vi "SSP - set cluster element.vi"(8 "error in (no error)":errorcluster, 11 "JSON string":string) -> (0 "error out":errorcluster, 3 "value":string)   [LabVIEW 2020, in "ui-testing.lvlib"]
doc: "copyright: Thomas Zilliox©"
uses:
  ui-testing.lvlib
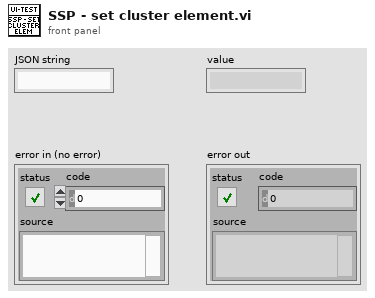
[diagram p1: front panel]
types:
  T1 = cluster{"name":string, "type":string, "value":string, "layers":string[], "subpanel":string, "subsubpanel":string}
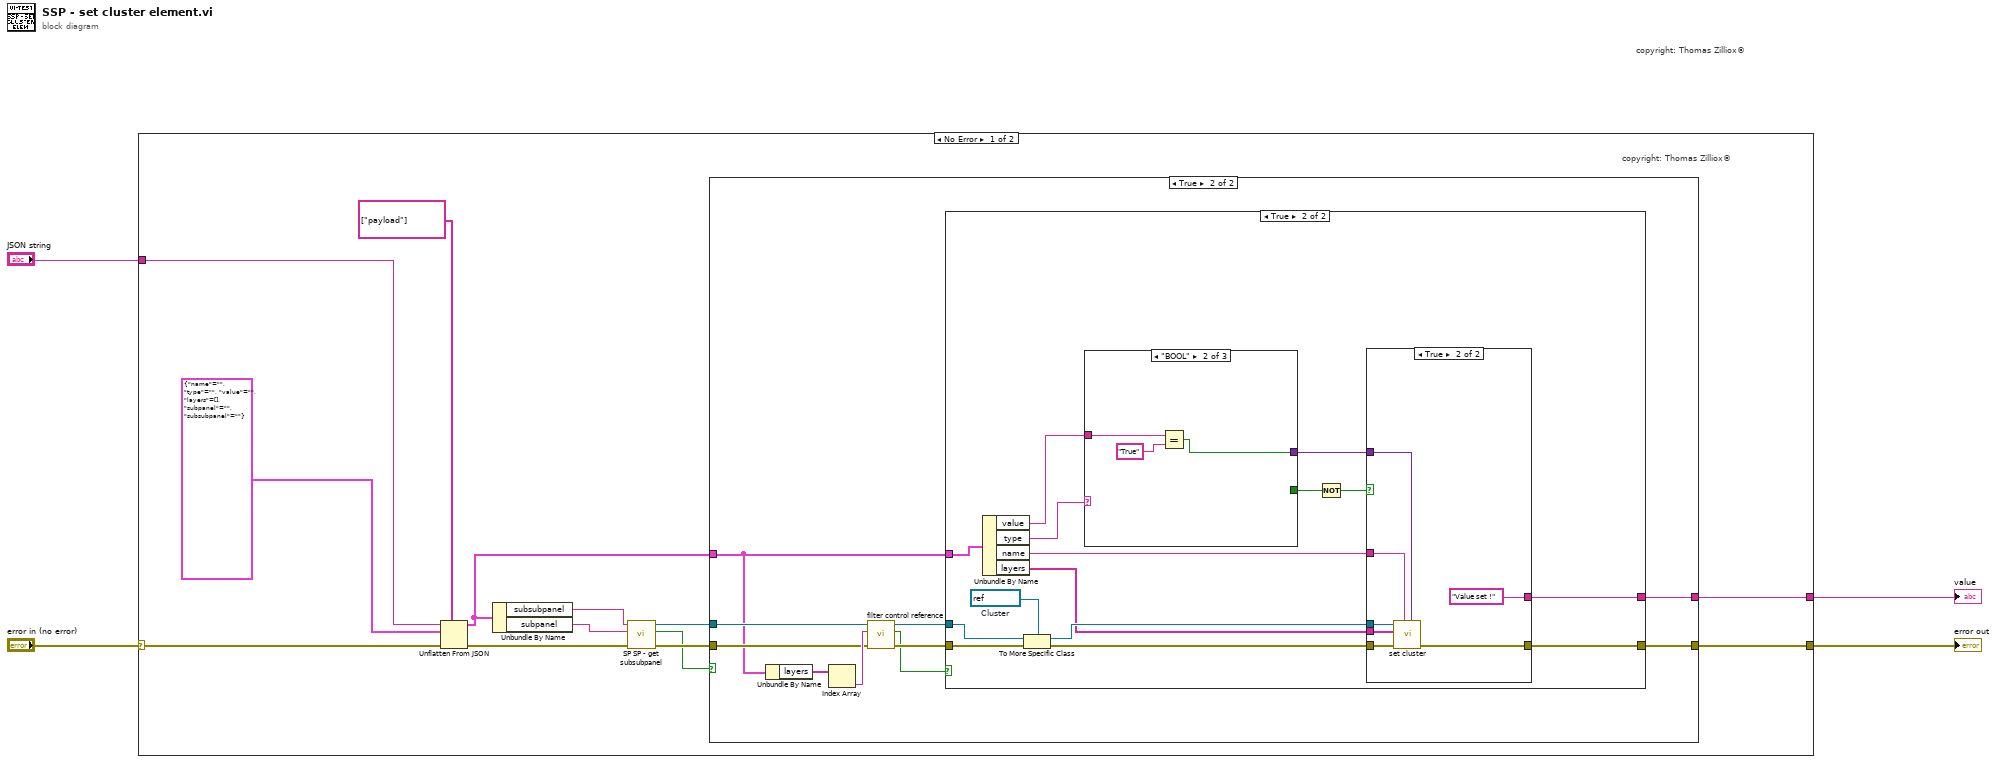
[diagram p0: block diagram]
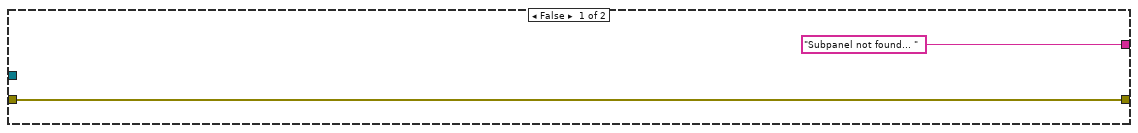
[diagram p2: hidden frame]
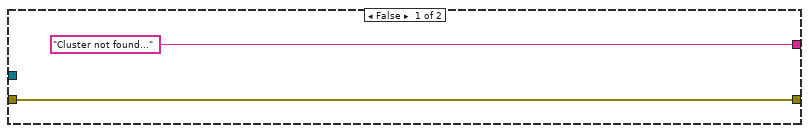
[diagram p3: hidden frame]
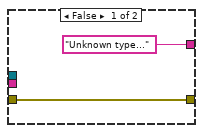
[diagram p4: hidden frame]
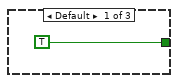
[diagram p5: hidden frame]
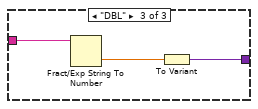
[diagram p6: hidden frame]
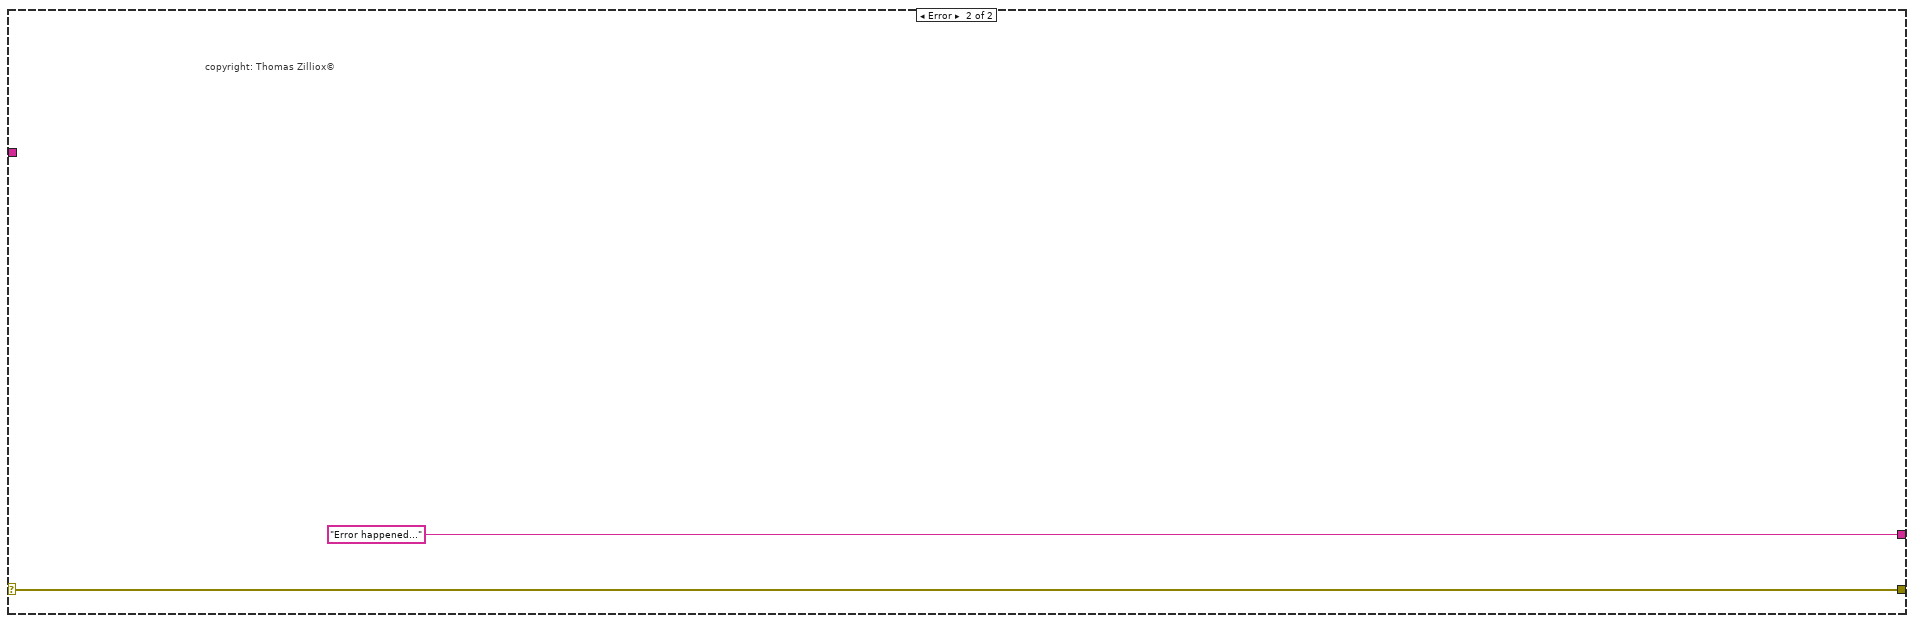
[diagram p7: hidden frame]
diagram:
  # "copyright: Thomas Zilliox©"
  n1 = case shown="No Error" "error in (no error)" {
    selector: "error in (no error)" -> [w15 w64]
    tunnel: "JSON string" -> [w16 _]
    tunnel: [w12 w64] -> w3
    tunnel: [w13 "Error happened..."] -> w2
    frame No Error {
      # "copyright: Thomas Zilliox©"
      n2 = Unflatten From JSON(path=string[] ["payload"], JSON string=w16, type and defaults=T1 {"name"="", "type"="", "value"="", "layers"=[], "subpanel"="", "subsubpanel"=""}, error in (no error)=w15) -> (value=w11:T1, error out=w8:errorcluster)  [unwired: 3 in]
      n3 = Unbundle By Name(w11) -> ("subsubpanel"=w10:string, "subpanel"=w9:string)
      n4 = call "SP SP - get subsubpanel.vi"("error in (no error)"=w8, "subpanel"=w9, "subsubpanel"=w10) -> ("error out"=w6:errorcluster, "SubSubPanel found"=w5:bool, "SubSubPanel VI"=w7:refnum<vi>)  [unwired: 5 in, 1 out]
      n5 = case shown="True" w5 {
        tunnel: ["Subpanel not found... " ("result string") w24] -> w13
        tunnel: [w18 w23] -> w12
        tunnel: w6 -> [w18 w22]
        tunnel: w7 -> [_ w21]
        tunnel: w11 -> [_ w20]
        frame False {
        }
        frame True {
          n6 = Unbundle By Name(w20) -> ("layers"=w29:string[])
          n7 = Index Array(array=w29) -> (element=w28:string)  [unwired: 1 in]
          n8 = call "filter control reference.vi"("error in (no error)"=w22, "Control label"=w28, "VI (Caller)"=w21) -> ("error out"=w26:errorcluster, "Control found"=w25:bool, "Control ref"=w27:refnum<vi>)  [unwired: 6 in]
          n9 = case shown="True" w25 {
            tunnel: w27 -> [_ w43]
            tunnel: w26 -> [w31 w46]
            tunnel: [w31 w45] -> w23
            tunnel: ["Cluster not found..." w34] -> w24
            tunnel: w20 -> [_ w40]
            frame False {
            }
            frame True {
              w41 = refnum<vi> refnum  # Cluster
              n10 = Unbundle By Name(w40) -> ("value"=w33:string, "type"=w37:string, "name"=w38:string, "layers"=w39:string[])
              n11 = To More Specific Class(target class=w41, reference=w43, error in=w46) -> (specific class reference=w42:refnum<vi>, error out=w44:errorcluster)
              n12 = case shown="\"BOOL\"" w37 {
                tunnel: [TRUE _ _] -> w36
                tunnel: [_ w57 w62] -> w32
                tunnel: w33 -> [_ w59 w61]
                frame Default {
                }
                frame "BOOL" {
                  n13 = Equal?(x=w59, y="True") -> (x = y?=w57:bool)
                }
                frame "DBL" {
                  n14 = Fract/Exp String To Number(string=w61) -> (number=w60:dbl)  [unwired: 3 in, 1 out]
                  n15 = To Variant(anything=w60) -> (Variant=w62:variant)
                }
              }
              n16 = Not(x=w36) -> (.not. x?=w35:bool)
              n17 = case shown="True" w35 {
                tunnel: [w48 w55] -> w45
                tunnel: w44 -> [w48 w54]
                tunnel: w42 -> [_ w53]
                tunnel: w39 -> [_ w52]
                tunnel: w38 -> [_ w51]
                tunnel: ["Unknown type..." "Value set !"] -> w34
                tunnel: w32 -> [_ w49]
                frame False {
                }
                frame True {
                  n18 = call "set cluster.vi"("Value"=w49, "Label"=w51, "error in (no error)"=w54, "Layer arrary"=w52, "cluster ref"=w53) -> ("error out"=w55:errorcluster)  [unwired: 6 in]
                }
              }
            }
          }
        }
      }
    }
    frame Error {
      # "copyright: Thomas Zilliox©"
    }
  }
  "error out" <- w3
  "value" <- w2
